vi "CIF Template UI _orig.vi"() -> ()   [LabVIEW 2021, in "CIF Template UI.lvlib"]
uses:
  CIF Template UI.lvlib
  CIF-LVCore/src/CIFUI/Typedef/Channel Connection.ctl
  CIF-LVCore/src/CIFUI/Typedef/Force Channel.ctl
  CIF-LVCore/src/CIFUI/Typedef/Run Listen Button.ctl
  Common/Typedef/Configuration.ctl
  CIF-LVCore/src/CIFCore/Common/Typedef/Common Plugin Configuration.ctl
  CIF-LVCore/src/CIFUI/Typedef/Core UI References.ctl
  CIF-LVCore/src/CIFUI/CIF_UI.lvclass/CIF_UI.ctl
  CIF-LVCore/src/CIFUI/Typedef/Direction to Include.ctl
  CIF-LVCore/src/CIFUI/UI Element Update/Empty Tree by Reference.vi
  CIF-LVCore/src/CIFUI/UI Element Update/Empty Table by Reference.vi
  CIF-LVCore/src/CIFUI/UI Element Update/Initialize Manager Tab by Reference.vi
  CIF-LVCore/src/CIFUI/CIF_UI.lvclass
  <vilib>/addons/_JKI.lib/Serialization/JSON/JKI JSON Serialization.lvlib
  Grpc/Template_wrapper/TemplateWrapper.lvlib
  CIF-LVCore/src/CIFCore/Common/CIFCoreCommon.lvlib
  Common/TemplateCommon.lvlib
panel:
  in  "Plugin Status":string[][](table)
  in  "Configuration":T1={"Common"={"Period (s)"=0.001, "Offset (us)"=0, "ClockID"=0, "Priority"=100, "Processor"=-2}, "Step"=100} {"Common"."Period (s)" format="%#_13g"}
  out "Errors":string
  in  "Run Listen":T3
  in  "Exit":bool
  out "Connected":bool
  in  "Connection":bool
  in  "Force Channel":T4
  in  "Link Channel":bool
  in  "Connection":T5
  in  "Channels":string(tree)
  in  "address":string="192.168.1.160"
  in  "Clear Local":bool
  in  "Force":bool
  in  "Unload":bool
  in  "Refresh Button":bool
  in  "Update Config":bool
  in  "Session Id":u64
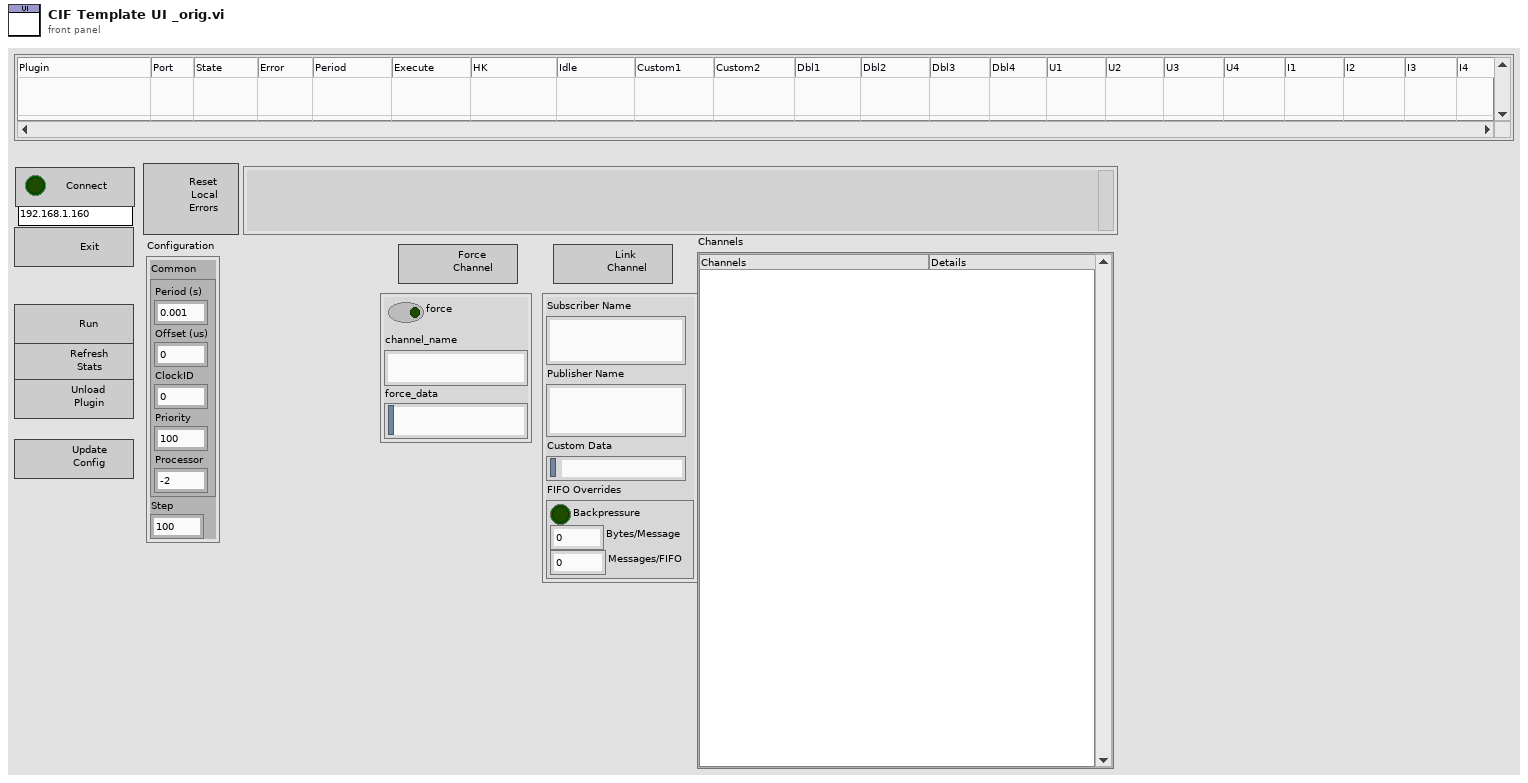
[diagram p1: front panel]
types:
  T1 = typedef "TemplateCommon.lvlib/Configuration.ctl" = cluster{"Common":T2, "Step":u64}
  T2 = typedef "CIFCoreCommon.lvlib/Common Plugin Configuration.ctl" = cluster{"Period (s)":dbl, "Offset (us)":i32, "ClockID":u8, "Priority":i32, "Processor":i32}
  T3 = typedef "CIF_UI.lvclass/Run Listen Button.ctl" = bool
  T4 = typedef "CIF_UI.lvclass/Force Channel.ctl" = cluster{"channel_name":string, "force":bool, "force_data":string}
  T5 = typedef "CIF_UI.lvclass/Channel Connection.ctl" = cluster{"Subscriber Name":string, "Publisher Name":string, "Custom Data":string, "FIFO Overrides":cluster{"Backpressure":bool, "Bytes/Message":u32, "Messages/FIFO":u32}}
  T6 = typedef "CIF_UI.lvclass/Core UI References.ctl" = cluster{"Discovered Plugins":refnum<vi>, "Discovered Plugins Valid":bool, "Loaded Plugins":refnum<vi>, "Loaded Plugins Valid":bool, "Publisher Channels":refnum<vi>, "Publisher Channels Valid":bool, "Subscriber Channels":refnum<vi>, "Subscriber Channels Valid":bool, "Plugin Status":refnum<vi>, "Plugin Status Valid":bool, "Channel Connection":refnum<vi>, "Channel Connection Valid":bool, "New Plugin Load":refnum<vi>, "New Plugin Load Valid":bool, "Errors":refnum<vi>, "Errors Valid":bool, "Plugin to Abort":refnum<vi>, "Plugin to Abort Valid":bool, "Connection":refnum<vi>, "Connection Valid":bool, "Exit":refnum<vi>, "Exit Valid":bool, "Run Listen":refnum<vi>, "Run Listen Valid":bool, "CIF Manager Tab":refnum<vi>, "Manger Tab Valid":bool, "Clear Local Error":refnum<vi>, "Clear Local Error Valid":bool, "Local Error":refnum<vi>, "Local Error Valid":bool, "System Errors":refnum<vi>, "System Errors Valid":bool, "Plugin Selection":refnum<vi>, "Plugin Selection Valid":bool}
  T7 = typedef "InstrumentStudio Plugin SDK.lvlib/Event Registration Refnum.ctl" = refnum<event-registration>
  T8 = typedef "CIF_UI.lvclass/Direction to Include.ctl" = enum16{"All", "Subscriber", "Publisher"}
  T9 = typedef "grpc-lvsupport-release.lvlib/grpcId.ctl" = u64
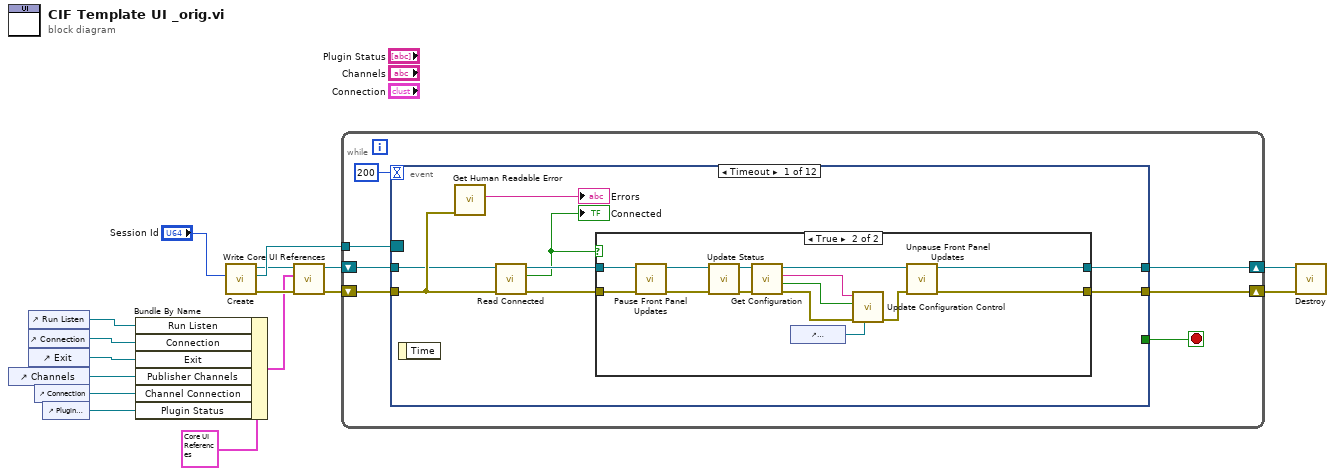
[diagram p0: block diagram]
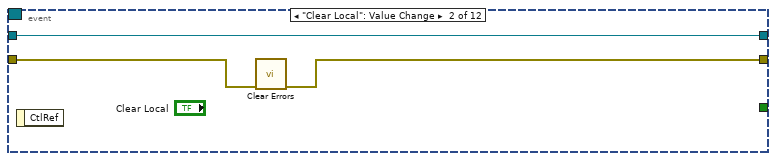
[diagram p3: hidden frame]
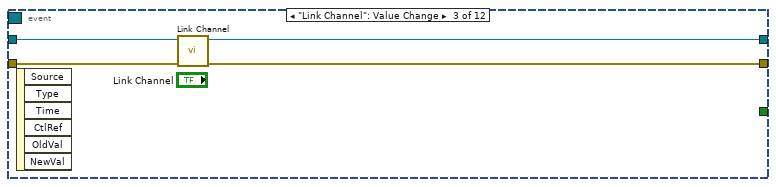
[diagram p4: hidden frame]
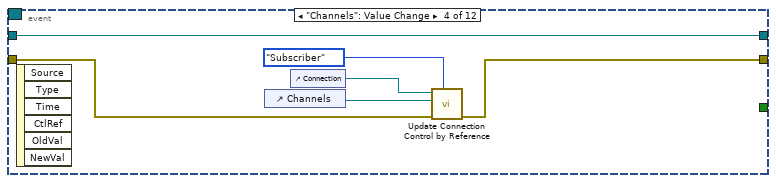
[diagram p5: hidden frame]
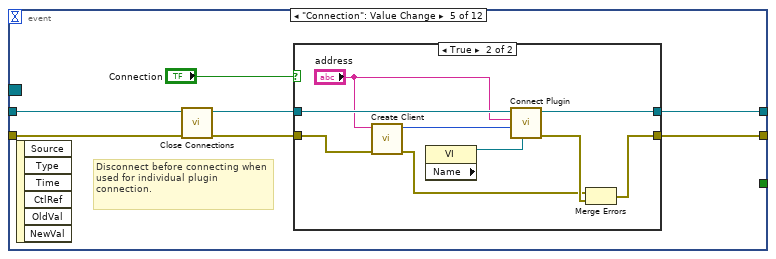
[diagram p6: hidden frame]
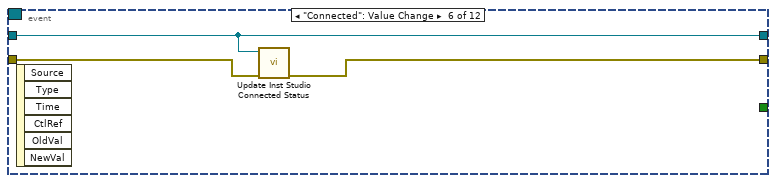
[diagram p8: hidden frame]
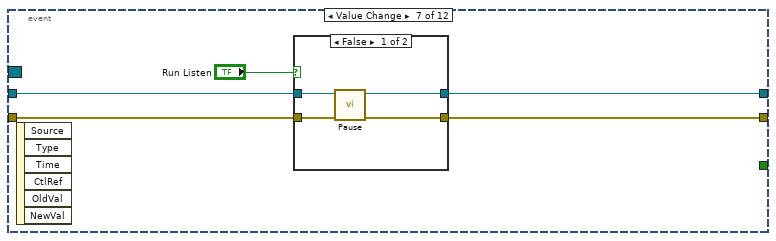
[diagram p9: hidden frame]
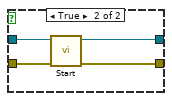
[diagram p10: hidden frame]
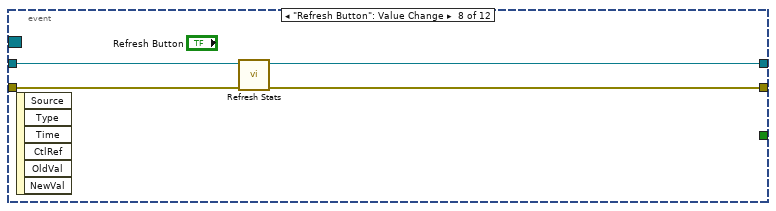
[diagram p11: hidden frame]
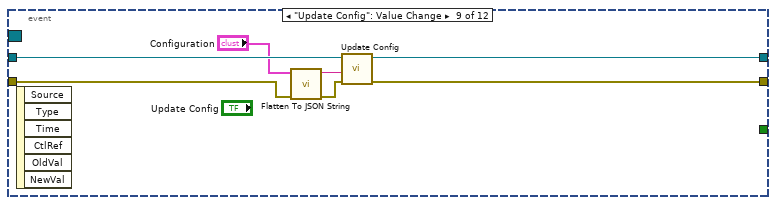
[diagram p12: hidden frame]
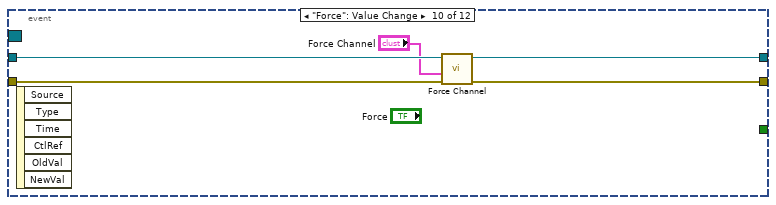
[diagram p13: hidden frame]
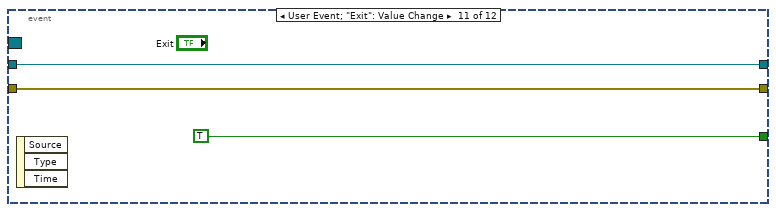
[diagram p14: hidden frame]
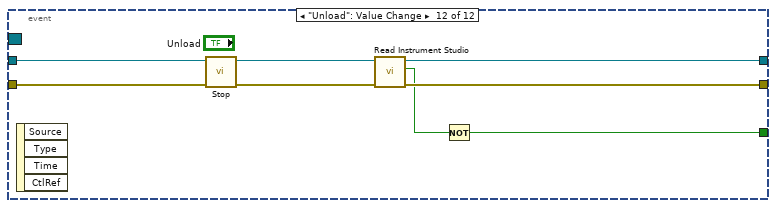
[diagram p15: hidden frame]
diagram:
  n1 = control-ref of="Channels"() -> (w14:refnum<vi>)
  n2 = control-ref of="Run Listen"() -> (w3:refnum<vi>)
  n3 = control-ref of="Connection"() -> (w4:refnum<vi>)
  n4 = control-ref of="Exit"() -> (w5:refnum<vi>)
  n5 = control-ref of="Connection"() -> (w2:refnum<vi>)
  n6 = control-ref of="Plugin Status"() -> (w1:refnum<vi>)
  n7 = Bundle By Name(cluster=T6 {"Discovered Plugins"=refnum, "Discovered Plugins Valid"=FALSE, "Loaded Plugins"=refnum, "Loaded Plugins Valid"=FALSE, "Publisher Channels"=refnum, "Publisher Channels Valid"=FALSE, "Subscriber Channels"=refnum, "Subscriber Channels Valid"=FALSE, "Plugin Status"=refnum, "Plugin Status Valid"=FALSE, "Channel Connection"=refnum, "Channel Connection Valid"=FALSE, "New Plugin Load"=refnum, "New Plugin Load Valid"=FALSE, "Errors"=refnum, "Errors Valid"=FALSE, "Plugin to Abort"=refnum, "Plugin to Abort Valid"=FALSE, "Connection"=refnum, "Connection Valid"=FALSE, "Exit"=refnum, "Exit Valid"=FALSE, "Run Listen"=refnum, "Run Listen Valid"=FALSE, "CIF Manager Tab"=refnum, "Manger Tab Valid"=FALSE, "Clear Local Error"=refnum, "Clear Local Error Valid"=FALSE, "Local Error"=refnum, "Local Error Valid"=FALSE, "System Errors"=refnum, "System Errors Valid"=FALSE, "Plugin Selection"=refnum, "Plugin Selection Valid"=FALSE} ("UI References"), "Run Listen"=w3, "Connection"=w4, "Exit"=w5, "Publisher Channels"=w14, "Channel Connection"=w2, "Plugin Status"=w1) -> (w7:T6)
  n8 = call "Create.vi"("Session Id"="Session Id") -> ("error out"=w10:errorcluster, "Event Refnum"=w13:T7, "CIF_UI out"=w11:refnum<class "CIF_UI.lvclass">)  [unwired: 8 in]
  n9 = call "Write Core UI References.vi"("error in (no error)"=w10, "UI References"=w7, "CIF_UI in"=w11) -> ("error out"=w8:errorcluster, "CIF_UI out"=w9:refnum<class "CIF_UI.lvclass">)  [unwired: 7 in]
  n10 = while {
    tunnel: w13 -> [w22]
    shift-right: [w17] -> w15
    shift-left: w9 -> [w20]
    shift-right: [w18] -> w16
    shift-left: w8 -> [w19]
    stop <- w21 stop-if-true
    n11 = event shown="[0] Timeout" {
      selector: w22 -> [_ _ _ _ _ _ _ _ _ _ _ _]
      dyn-events: _ -> [_ _ _ _ _ _ _ _ _ _ _ _]
      timeout: 200 -> [_ _ _ _ _ _ _ _ _ _ _ _]
      tunnel: [_ _ _ _ _ _ _ _ _ _ TRUE w114] -> w21
      tunnel: w20 -> [w24 w48 w54 w55 w65 w79 w85 w98 w105 w110 w112 w121]
      tunnel: w19 -> [w25 w50 w53 w57 w64 w81 w86 w97 w101 w109 w111 w120]
      tunnel: [w27 w49 w52 w56 w67 w80 w83 w96 w103 w107 w111 w116] -> w18
      tunnel: [w31 w48 w51 w55 w66 w79 w84 w95 w104 w108 w112 w117] -> w17
      event Timeout {
        n12 = event-data() -> ()  [unwired: 1 in, 1 out]
        n13 = call "Get Human Readable Error.vi"("error in (no error)"=w25) -> ("Error Message"=→"Errors":string)  [unwired: 10 in]
        n14 = call "Read Connected.vi"("error in (no error)"=w25, "CIF_UI in"=w24) -> ("error out"=w29:errorcluster, "Connected"=w28:bool, "CIF_UI out"=w30:refnum<class "CIF_UI.lvclass">)  [unwired: 7 in]
        "Connected" <- w28
        n15 = case shown="True" w28 {
          tunnel: w29 -> [w32 w44]
          tunnel: [w32 w47] -> w27
          tunnel: w30 -> [w33 w45]
          tunnel: [w33 w46] -> w31
          frame False {
          }
          frame True {
            n16 = call "Pause Front Panel Updates.vi"("error in (no error)"=w44, "CIF_UI in"=w45) -> ("error out"=w43:errorcluster, "CIF_UI out"=w42:refnum<class "CIF_UI.lvclass">)  [unwired: 8 in]
            n17 = call "Update Status.vi"("error in (no error)"=w43, "CIF_UI in"=w42) -> ("error out"=w40:errorcluster, "CIF_UI out"=w41:refnum<class "CIF_UI.lvclass">)  [unwired: 8 in]
            n18 = call "Get Configuration.vi"("error in (no error)"=w40, "CIF_Plugin_UI in"=w41) -> ("error out"=w38:errorcluster, "Not Found"=w35:bool, "JSON Configuration"=w36:string, "CIF_Plugin_UI out"=w39:refnum<class "CIF_UI.lvclass">)  [unwired: 6 in]
            n19 = control-ref of="Configuration"() -> (w34:refnum<vi>)
            n20 = call "Update Configuration Control.vi"("Configuration reference"=w34, "error in (no error)"=w38, "Not Valid"=w35, "JSON Configuration"=w36) -> ("error out"=w37:errorcluster)  [unwired: 7 in]
            n21 = call "Unpause Front Panel Updates.vi"("error in (no error)"=w37, "CIF_UI in"=w39) -> ("error out"=w47:errorcluster, "CIF_UI out"=w46:refnum<class "CIF_UI.lvclass">)  [unwired: 8 in]
          }
        }
      }
      event "Clear Local": Value Change {
        n22 = event-data() -> ()  [unwired: 1 in, 1 out]
        n23 = call <vilib>:"Clear Errors.vi"("error in (no error)"=w50) -> ("error out"=w49:errorcluster)  [unwired: 5 in, 1 out]
      }
      event "Link Channel": Value Change {
        n24 = event-data() -> ()  [unwired: 1 in, 6 out]
        n25 = call "Link Channel.vi"("error in (no error)"=w53, "CIF_UI in"=w54) -> ("error out"=w52:errorcluster, "CIF_UI out"=w51:refnum<class "CIF_UI.lvclass">)  [unwired: 8 in]
      }
      event "Channels": Value Change {
        n26 = event-data() -> ()  [unwired: 1 in, 6 out]
        n27 = control-ref of="Channels"() -> (w58:refnum<vi>)
        n28 = control-ref of="Connection"() -> (w59:refnum<vi>)
        n29 = call "Update Connection Control by Reference.vi"("Direction to Include"=Direction_to_Include."Subscriber", "error in (no error)"=w57, "Channels"=w58, "Channel Connection"=w59) -> ("error out"=w56:errorcluster)  [unwired: 6 in, 1 out]
      }
      event "Connection": Value Change {
        # "Disconnect before connecting when used for individual plugin connection."
        n30 = event-data() -> ()  [unwired: 1 in, 6 out]
        n31 = call "Close Connections.vi"("error in (no error)"=w64, "CIF_UI in"=w65) -> ("error out"=w62:errorcluster, "CIF_UI out"=w63:refnum<class "CIF_UI.lvclass">)  [unwired: 8 in]
        n32 = case shown="True" "Connection" {
          tunnel: [w68 w78] -> w67
          tunnel: [w69 w76] -> w66
          tunnel: w63 -> [w69 w75]
          tunnel: w62 -> [w68 w74]
          frame False {
          }
          frame True {
            n33 = call "Create Client.vi"("error in"=w74, "address"="address") -> ("error out"=w73:errorcluster, "gRPC ID Out"=w70:T9)  [unwired: 8 in]
            n34 = property class="VI" props=["Name"]() -> (reference out=w71:refnum<vi>)  [unwired: 2 in, 2 out]
            n35 = call "Connect Plugin.vi"("VI Reference"=w71, "gRPC ID"=w70, "Address"="address", "CIF_UI in"=w75) -> ("error out"=w77:errorcluster, "CIF_UI out"=w76:refnum<class "CIF_UI.lvclass">)  [unwired: 6 in]
            n36 = Merge Errors(w73, w77) -> (w78:errorcluster)
          }
        }
      }
      event "Connected": Value Change {
        n37 = event-data() -> ()  [unwired: 1 in, 6 out]
        n38 = call "Update Inst Studio Connected Status.vi"("error in (no error)"=w81, "CIF_UI in"=w79) -> ("error out"=w80:errorcluster)  [unwired: 9 in]
      }
      event Value Change {
        n39 = event-data() -> ()  [unwired: 1 in, 6 out]
        n40 = case shown="False" "Run Listen" {
          tunnel: w86 -> [w90 w94]
          tunnel: w85 -> [w89 w93]
          tunnel: [w87 w92] -> w84
          tunnel: [w88 w91] -> w83
          frame False {
            n41 = call "Pause.vi"("error in (no error)"=w90, "CIF_Plugin_UI in"=w89) -> ("error out"=w88:errorcluster, "CIF_Plugin_UI out"=w87:refnum<class "CIF_UI.lvclass">)  [unwired: 7 in, 1 out]
          }
          frame True {
            n42 = call "Start.vi"("error in (no error)"=w94, "CIF_Plugin_UI in"=w93) -> ("error out"=w91:errorcluster, "CIF_Plugin_UI out"=w92:refnum<class "CIF_UI.lvclass">)  [unwired: 7 in, 1 out]
          }
        }
      }
      event "Refresh Button": Value Change {
        n43 = event-data() -> ()  [unwired: 1 in, 6 out]
        n44 = call "Refresh Stats.vi"("error in (no error)"=w97, "CIF_Plugin_UI in"=w98) -> ("error out"=w96:errorcluster, "CIF_Plugin_UI out"=w95:refnum<class "CIF_UI.lvclass">)  [unwired: 7 in, 1 out]
      }
      event "Update Config": Value Change {
        n45 = event-data() -> ()  [unwired: 1 in, 6 out]
        n46 = call <vilib>:"Flatten To JSON String.vi"("error in (no error)"=w101, "Variant"="Configuration") -> ("error out"=w99:errorcluster, "JSON String"=w100:string)  [unwired: 8 in]
        n47 = call "Update Config.vi"("error in (no error)"=w99, "JSON Configuration"=w100, "CIF_Plugin_UI in"=w105) -> ("error out"=w103:errorcluster, "CIF_Plugin_UI out"=w104:refnum<class "CIF_UI.lvclass">)  [unwired: 6 in, 1 out]
      }
      event "Force": Value Change {
        n48 = event-data() -> ()  [unwired: 1 in, 6 out]
        n49 = call "Force Channel.vi"("error in (no error)"=w109, "Force Channel"="Force Channel", "CIF_Plugin_UI in"=w110) -> ("error out"=w107:errorcluster, "CIF_Plugin_UI out"=w108:refnum<class "CIF_UI.lvclass">)  [unwired: 6 in, 1 out]
      }
      event User Event; "Exit": Value Change {
        n50 = event-data() -> ()  [unwired: 1 in, 3 out]
      }
      event "Unload": Value Change {
        n51 = event-data() -> ()  [unwired: 1 in, 4 out]
        n52 = call "Stop.vi"("error in (no error)"=w120, "CIF_Plugin_UI in"=w121) -> ("error out"=w118:errorcluster, "CIF_Plugin_UI out"=w119:refnum<class "CIF_UI.lvclass">)  [unwired: 7 in, 1 out]
        n53 = call "Read Instrument Studio.vi"("error in (no error)"=w118, "CIF_UI in"=w119) -> ("error out"=w116:errorcluster, "Instrument Studio"=w115:bool, "CIF_UI out"=w117:refnum<class "CIF_UI.lvclass">)  [unwired: 7 in]
        n54 = Not(x=w115) -> (.not. x?=w114:bool)
      }
    }
  }
  n55 = call "Destroy.vi"("error in (no error)"=w16, "CIF_UI in"=w15) -> ()  [unwired: 8 in, 2 out]
